vi "Auton List.vi"() -> (3 "String Array":string[](array[string]))   [LabVIEW 2018]
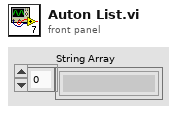
[diagram p1: front panel]
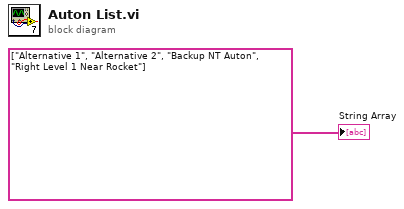
[diagram p0: block diagram]
diagram:
  "String Array" <- string[] ["Alternative 1", "Alternative 2", "Backup NT Auton", "Right Level 1 Near Rocket"] ("String Array")
